vi "Read Singel Item.vi"(8 "Tag":string, 10 "Parent Tag":string, 11 "Tree in":refnum<class "Tree.lvclass">) -> (2 "Element Out":T1, 3 "Tree out":refnum<class "Tree.lvclass">)   [LabVIEW 2024, in "Tree.lvclass"]
doc: "This VI will Fill the Single Item \nWith The Input Tag Item\n\nThe Parent Will Be Searched\nIF the Input \"Parent Tag\"\nWasn't Connected"
uses:
  Tree.lvclass
  Type Def/Tree Item.ctl
  Tree.lvclass/Tree.ctl
  Polymorphic VIs/Tree Converter/Tag To BFS Index.vi
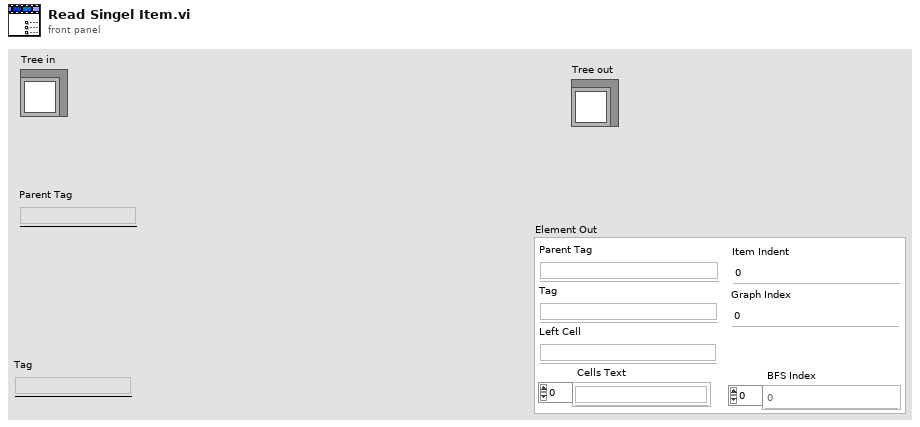
[diagram p1: front panel]
types:
  T1 = typedef "Tree Item.ctl" = cluster{"Parent Tag":string, "Tag":string, "Left Cell":string, "Cells Text":string[], "BFS Index":i32[], "Graph Index":i32, "Item Indent":i32}
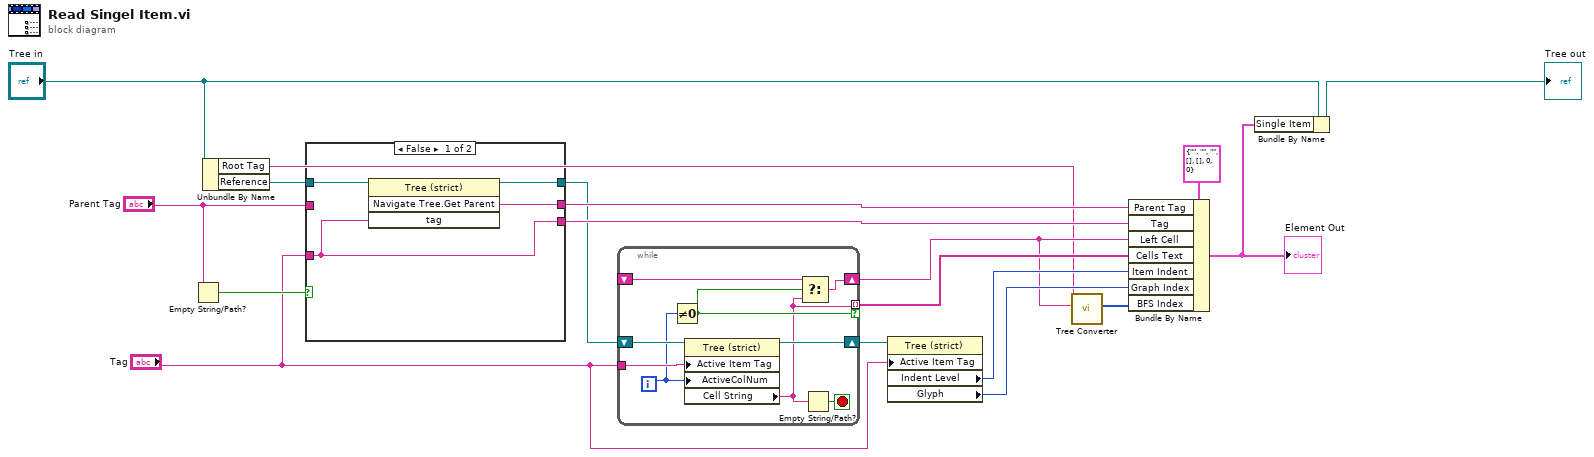
[diagram p0: block diagram]
diagram:
  n1 = Empty String/Path?(string/path="Parent Tag") -> (empty?=w16:bool)
  n2 = Unbundle By Name("Tree in") -> ("Root Tag"=w1:string, "Reference"=w17:refnum<vi>)
  n3 = case shown="False" w16 {
    tunnel: w17 -> [w22 w23]
    tunnel: "Parent Tag" -> [_ w25]
    tunnel: [w21 w25] -> w15
    tunnel: "Tag" -> [w19 w24]
    tunnel: [w20 w23] -> w13
    tunnel: [w19 w24] -> w14
    frame False {
      n4 = invoke class="Tree (strict)" method="Navigate Tree.Get Parent"(reference=w22, "tag"=w19) -> (reference out=w20:refnum<vi>, "Navigate Tree:Get Parent"=w21:string)  [unwired: 2 in, 2 out]
    }
    frame True {
    }
  }
  n5 = while {
    tunnel: "Tag" -> [w33]
    shift-right: [w32] -> w11
    shift-left: w13 -> [w34]
    tunnel: [w28] -> w12 mode=indexing if=w29
    shift-right: [w27] -> w3
    shift-left: _ -> [w26]
    i -> [w31]
    stop <- w30 stop-if-true
    n6 = Not Equal To 0?(x=w31) -> (x != 0?=w29:bool)
    n7 = property class="Tree (strict)"(reference=w34, "Active Item Tag"=w33, "ActiveColNum"=w31) -> (reference out=w32:refnum<vi>, "Cell String"=w28:string)  [unwired: 1 in, 1 out]
    n8 = Select(t=w26, s=w29, f=w28) -> (s? t:f=w27:string)
    n9 = Empty String/Path?(string/path=w28) -> (empty?=w30:bool)
  }
  n10 = property class="Tree (strict)"(reference=w11, "Active Item Tag"="Tag") -> ("Indent Level"=w10:i32, "Glyph"=w9:i32)  [unwired: 1 in, 2 out]
  n11 = call-poly "Tree Converter.vi"("Tag In"=w3, "Root Tag"=w1) -> ("BFS Index Out"=w2:i32[])  [unwired: 9 in]
  n12 = Bundle By Name(cluster=T1 {"Parent Tag"="", "Tag"="", "Left Cell"="", "Cells Text"=[], "BFS Index"=[], "Graph Index"=0, "Item Indent"=0} ("TreeItem"), "Parent Tag"=w15, "Tag"=w14, "Left Cell"=w3, "Cells Text"=w12, "Item Indent"=w10, "Graph Index"=w9, "BFS Index"=w2) -> (w7:T1)
  "Element Out" <- w7
  n13 = Bundle By Name(cluster="Tree in", "Single Item"=w7) -> (→"Tree out":refnum<class "Tree.lvclass">)
